vi "AMC_LabVIEW_GUI_Examle_.vi"() -> ()   [LabVIEW 2016]
uses:
  amc_api.lvlib
panel:
  in  "stop":bool
  in  "Tab Control":enum32{"Navigation", "Interface", "About"}(tab)
  out "MoveSignal":bool caption="Moving"
  out "Connected":bool=TRUE
  out "EotrightDetected1":bool caption="Status Eot FWD"
  out "EotLeftDetected1":bool caption="Status Eot BWD"
  out "move out":bool=TRUE caption="Move"
  out "in target range1":bool
  in  "Reset Error":bool
  out "Error":bool
  out "Error Message":string
  in  "Axis Tab Control":enum32{"Operation", "Settings"}(tab)
  out "R [Ohm]":i32
  out "C [nF]":i32
  in  "Single Step\nLeft":bool caption="Open Loop Funktions"
  in  "Single Step\nRight":bool caption="Step(s)"
  in  "Continuous Forward 2":bool caption="Continuous\nForward"
  in  "Endless Left":bool caption="Continuous\nBackward"
  in  "Amplitude [mV]":i32=45
  in  "Frequency [mHz]":i32=1999
  in  "Fixed DC 1":i32 caption="DC Level [mV]"
  in  "Axis 1":bool caption="Closed Loop Functions"
  out "Position":dbl=14701.126 caption="Position [nm]" format="%#_6f"
  out "ReferenceSignal":bool=TRUE
  in  "measureC&R":bool
  in  "Target Position 1":dbl caption="Target position [nm]"
  in  "Move 2":bool
  in  "Positioner":u16(ring)=15 items=["ANGp101", "ANGp50", "ANGt101", "ANGt51", "ANPx101", "ANPx311", "ANPx312", "ANPx321", "ANPx341", "ANPx51", "ANPz101", "ANPz101eXT", "ANPz102", "ANPz51", "ANPz51eXT", "ANR101", "ANR240", "ANR31", "ANR51", "ANRv220", "SNPopenLoop", "SNPxyBottom", "SNPxyTop"]
  in  "Number of steps":i32=1 caption="Number of Steps"
  in  "stop_on_EoT":bool caption="Stop on end of travel"
  in  "Target Range 1":i32 caption="Target Range [nm]"
  in  "Sensor Settings Tab Control":enum32{"NUM only", "RES only"}(tab)
  in  "auto Reset 1":bool=TRUE caption="Auto Reset"
  in  "Reference Auto Update 1":bool=TRUE caption="Auto update reference"
  in  "Configuration upload":path
  in  "Gound on target":bool
  in  "Sensor power":enum16{"0 dB", "-10 dB", "-15 dB", "-20 dB"}(ring)
  in  "auto measure C and R":bool
  in  "Disable Sensor":bool
  in  "Output":bool=TRUE caption="Axis 1"
  out "Output Status":bool=TRUE
  out "status":string
  out "RT Out Tab Control":enum32{"Off", "AquadB", "Trigger"}(tab)
  in  "AqaudB clock 1":i32 caption="AquadB Clock\n[ns], multiple of 40ns"
  in  "AquadB Resolution 1":i32 caption="AquadB\nResolution [nm]"
  in  "Trigger Config":T1
  out "Error 4":bool caption="Error"
  out "Error Message 4":string
  in  "Mode Input":u16(ring) caption="Mode" items=["Trigger (LVDS)"=11, "Trigger (LVTTL)"=10, "Stepper (LVDS)"=9, "Stepper (LVTTL)"=8, "AquadB (LVDS)"=1, "AquadB (LVTTL)"=0, "OFF"=15]
  in  "Loop Mode":u16(ring) caption="Loop mode" items=["closed-loop"=1, "open-loop"=0]
  in  "Steps per pulse":i32 caption="Steps per pulse [Steps]"
  in  "Change per pulse":i32 caption="Change per pulse [u°/nm]"
  in  "Reset Error 4":bool
  in  "Move":bool=TRUE
  in  "Signal mode":enum16{"LVTTL", "LVDS"}(ring)
  in  "RtOutMode":enum16{"Off", "AquadB", "Trigger"}(ring)
  in  "Reset Error 8":bool
  out "Error Message 7":string
  out "Error 7":bool caption="Error"
  out "Sn":string caption="Serial Number"
  out "ip":string="192.168.1.1" caption="IP Adress"
  out "Firmware Version":string
  out "Mac Adress":string
  out "authorized\nStatus":bool
  out "locked\nStatus":bool
  out "device name":string caption="Device Name"
  out "Device type":string="AMC100/NUM"
  out "Features acivated":string[](array[string])
  # "Individual Status Flags"
  # "Closed Loop Functions"
  # "(NUM only)"
  # "Diagnostic Tools (AMC300 only)"
  # "( /PRO Version only )"
  # "( /PRO Version only )"
  # "(AMC300 only)"
  # "Real Time Input"
  # "Real Time Output"
  # "Global Parameters"
  # "Axis 1"
  # "Axis 1"
  # "Device Info"
  # "Device Access"
  # "Features activated"
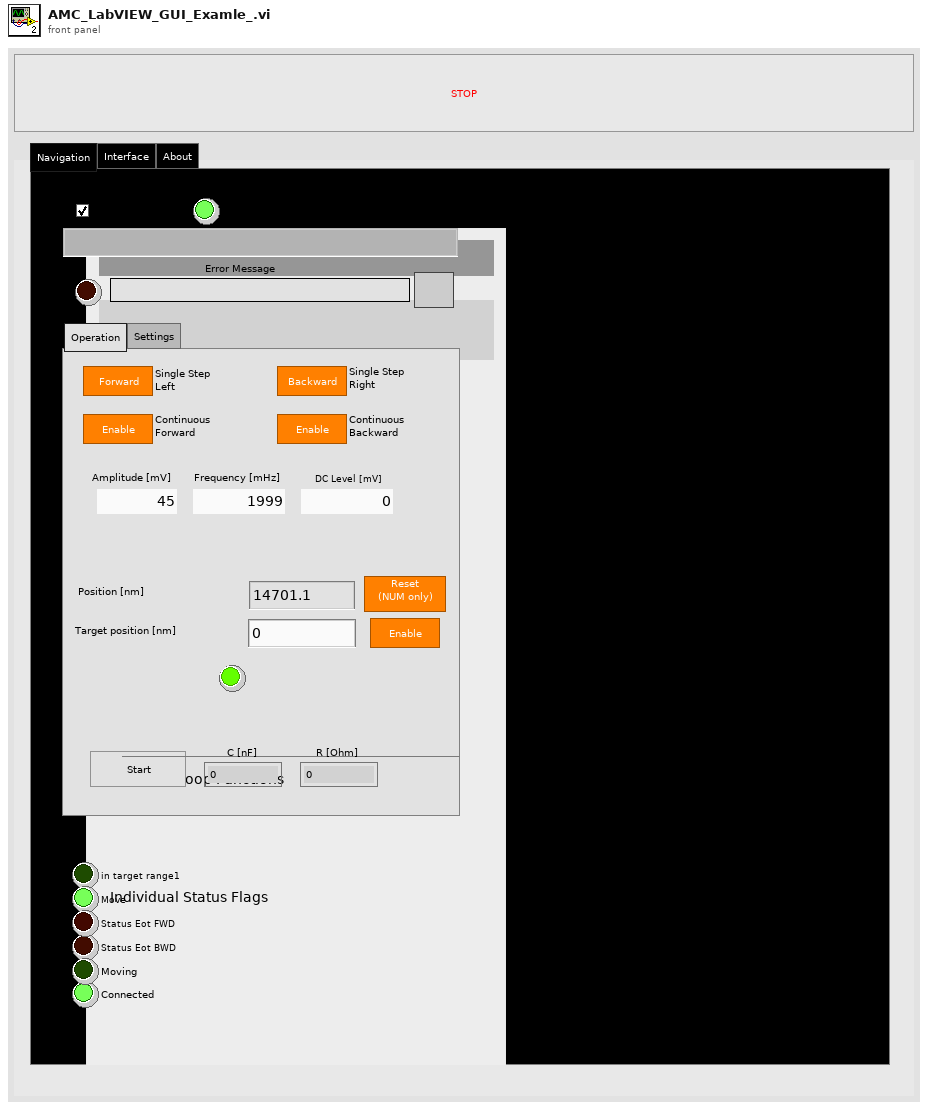
[diagram p1: front panel]
types:
  T1 = cluster{"Position high [nm]":i32, "Position low [nm]":i32, "Trigger polarity":enum16{"Active high", "Active low"}, "Epsilon [nm]":i32}
  T2 = enum8{"Enabled", "Disabled", "Disabled and Grayed Out"}
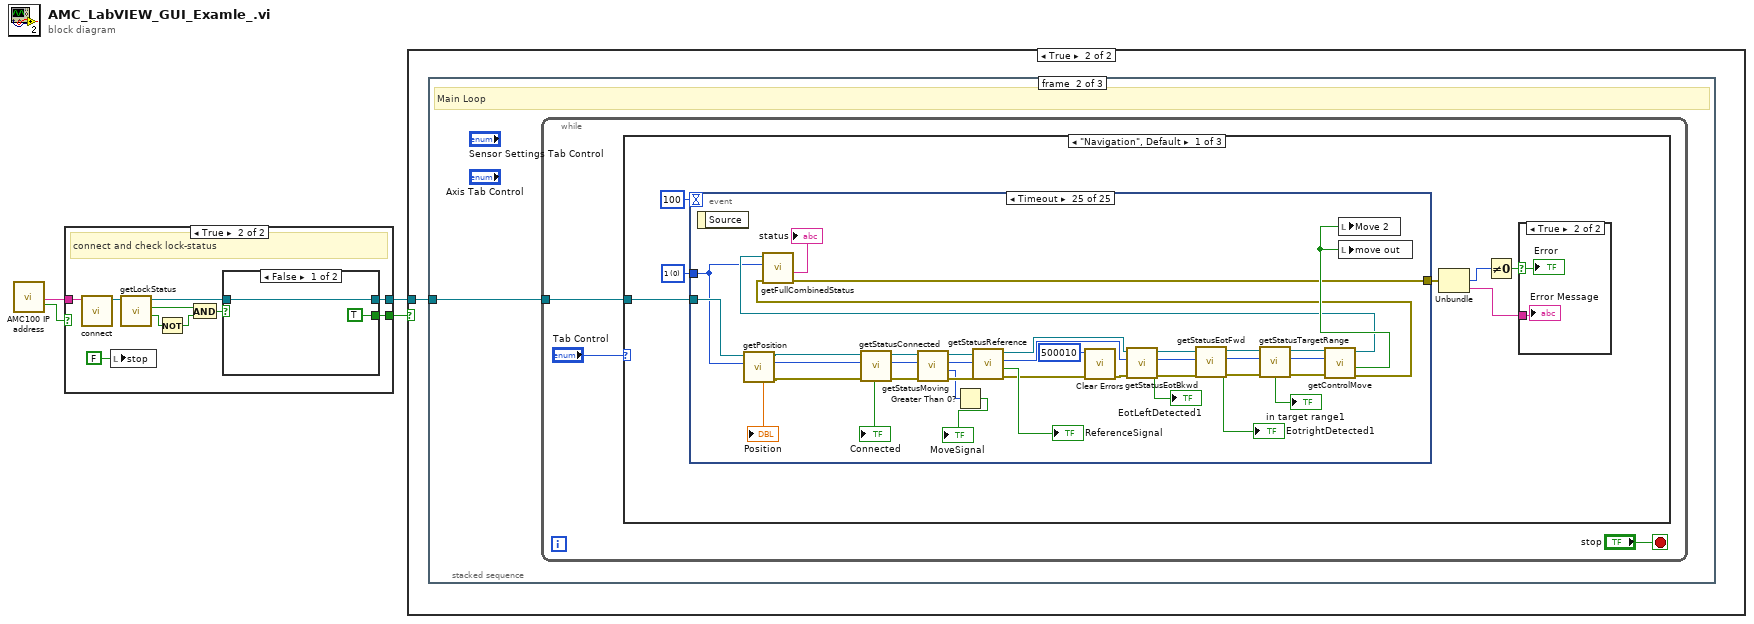
[diagram p0: block diagram]
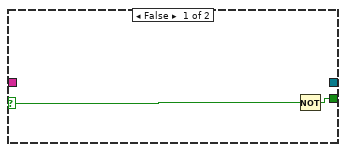
[diagram p2: hidden frame]
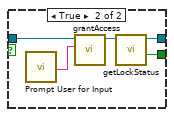
[diagram p3: hidden frame]
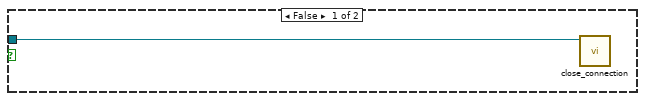
[diagram p4: hidden frame]
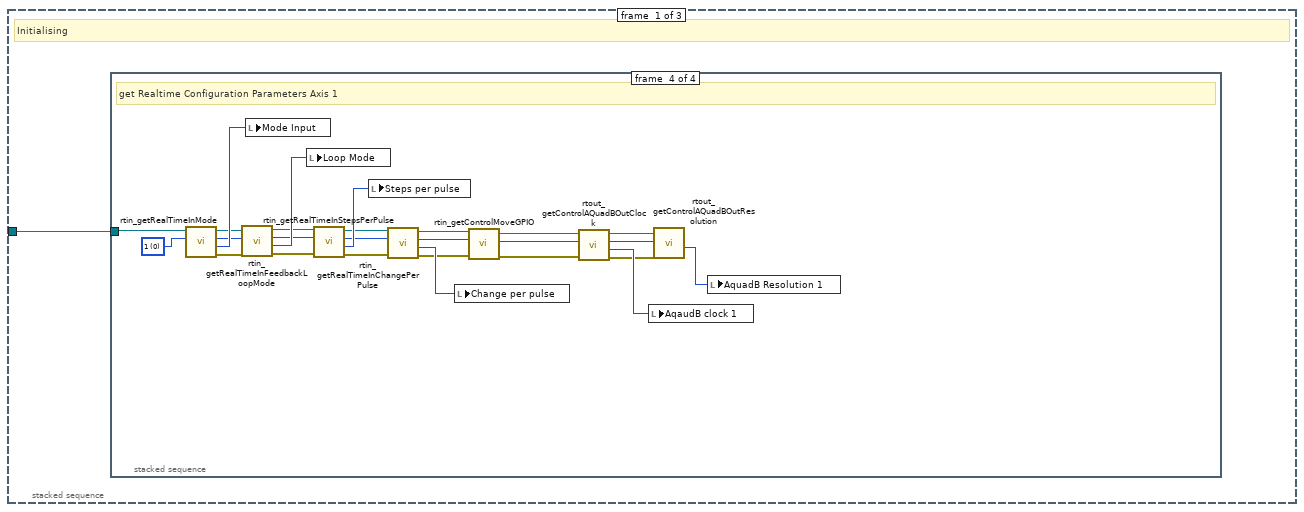
[diagram p5: hidden frame]
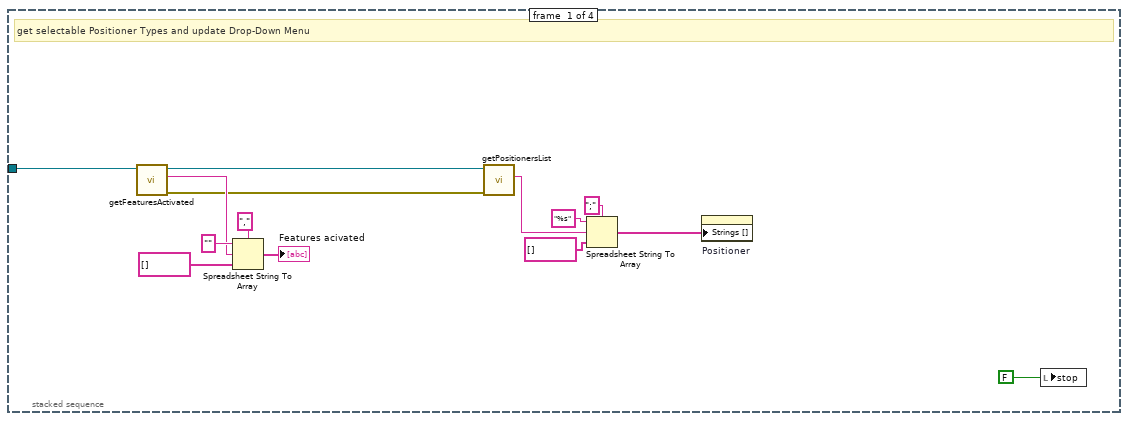
[diagram p6: hidden frame]
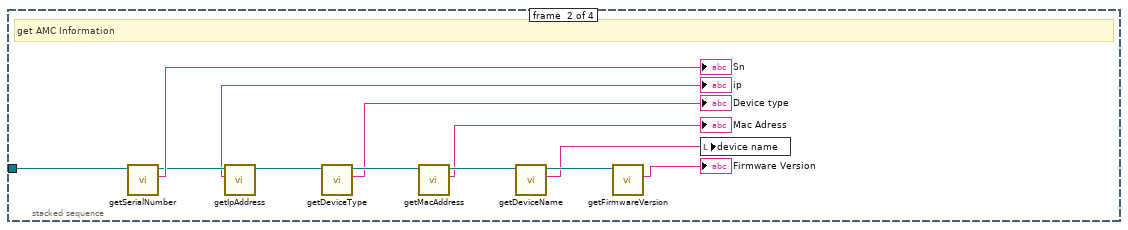
[diagram p7: hidden frame]
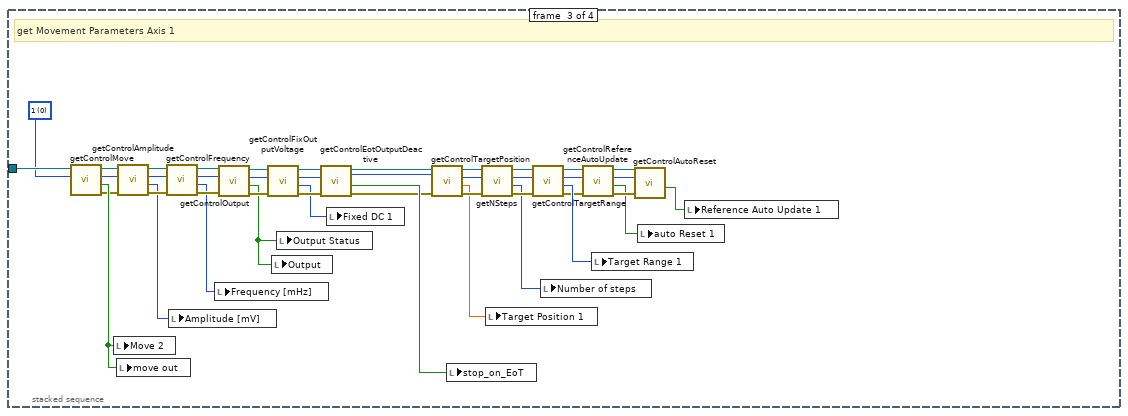
[diagram p8: hidden frame]
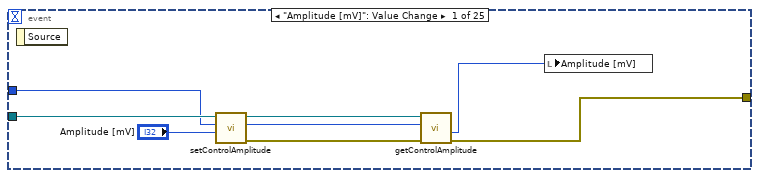
[diagram p10: hidden frame]
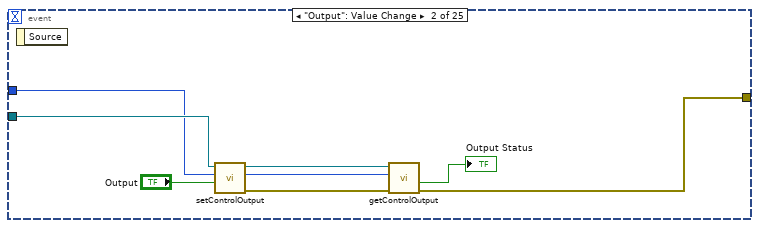
[diagram p11: hidden frame]
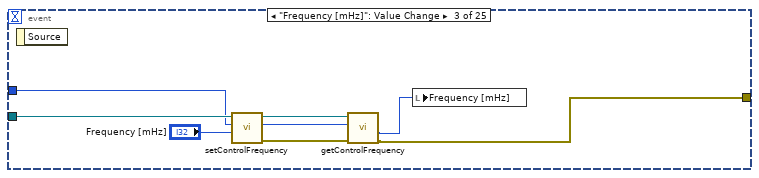
[diagram p12: hidden frame]
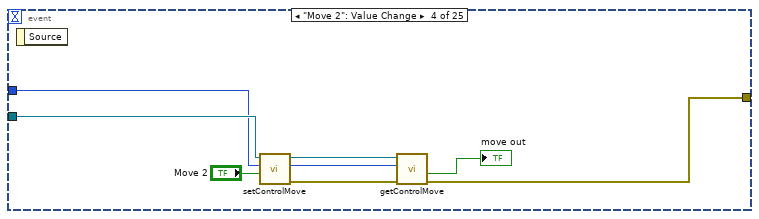
[diagram p13: hidden frame]
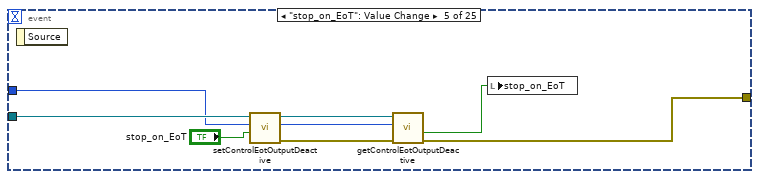
[diagram p14: hidden frame]
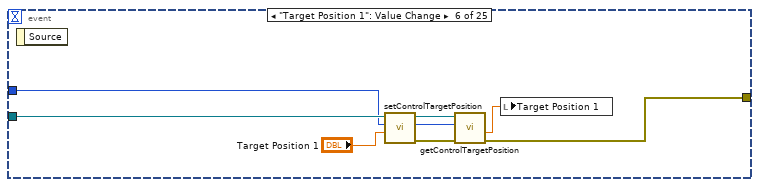
[diagram p15: hidden frame]
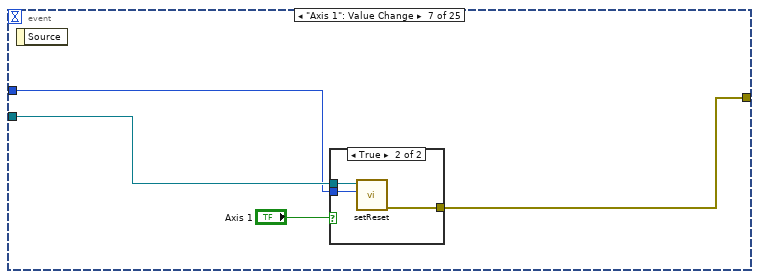
[diagram p16: hidden frame]
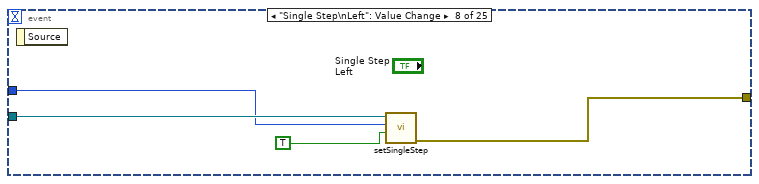
[diagram p18: hidden frame]
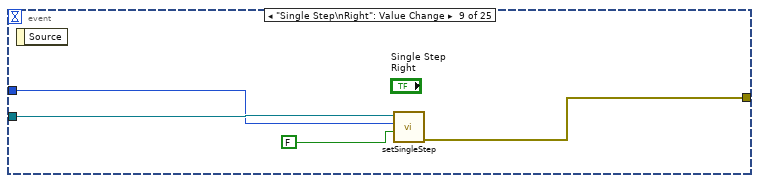
[diagram p19: hidden frame]
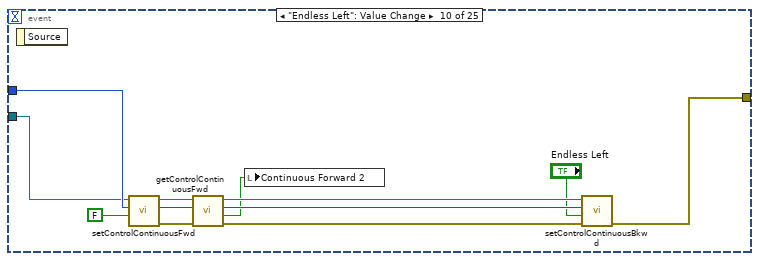
[diagram p20: hidden frame]
diagram:
  n1 = call "AMC100 IP address"() -> ("IP address"=w1:string, "OK"=w2:bool)  [unwired: 17 in, 1 out]
  n2 = case shown="True" w2 {
    selector: w2 -> [w5 _]
    tunnel: [w6 w16] -> w4
    tunnel: [_ w15] -> w3
    tunnel: w1 -> [_ w9]
    frame False {
      n3 = Not(x=w5) -> (.not. x?=w6:bool)
    }
    frame True {
      # "connect and check lock-status"
      n4 = call "connect.vi"("deviceAddress"=w9) -> ("connection ID"=w8:refnum<k5>)  [unwired: 5 in, 1 out]
      n5 = local write "stop"(FALSE ("stop")) -> ()
      n6 = call "getLockStatus.vi"("connection ID"=w8) -> ("authorized"=w11:bool, "locked"=w12:bool, "connection ID out"=w14:refnum<k5>)  [unwired: 7 in, 1 out]
      n7 = Not(x=w11) -> (.not. x?=w10:bool)
      n8 = And(x=w12, y=w10) -> (x .and. y?=w13:bool)
      n9 = case shown="False" w13 {
        tunnel: w14 -> [w18 w23]
        tunnel: [w18 w20] -> w15
        tunnel: [TRUE ("authorized") w19] -> w16
        frame False {
        }
        frame True {
          n10 = call "Prompt User for Input"() -> ("password"=w22:string)  [unwired: 17 in, 2 out]
          n11 = call "grantAccess.vi"("password"=w22, "connection ID"=w23) -> ("connection ID out"=w21:refnum<k5>)  [unwired: 8 in, 1 out]
          n12 = call "getLockStatus.vi"("connection ID"=w21) -> ("authorized"=w19:bool, "connection ID out"=w20:refnum<k5>)  [unwired: 7 in, 2 out]
        }
      }
    }
  }
  n13 = case shown="True" w4 {
    tunnel: w3 -> [w24 w25]
    frame False {
      n14 = call "close_connection.vi"("connection ID"=w24) -> ()  [unwired: 6 in, 1 out]
    }
    frame True {
      n15 = stacked-sequence {
        tunnel: w25 -> [w26 w122 w562]
        frame #0 {
          # "Initialising"
          n16 = stacked-sequence {
            tunnel: w26 -> [w39 w52 w63 w121]
            frame #0 {
              # "get selectable Positioner Types and update Drop-Down Menu"
              n17 = call "getFeaturesActivated.vi"("connection ID"=w39) -> ("error out"=w33:errorcluster, "features"=w36:string, "connection ID out"=w32:refnum<k5>)  [unwired: 8 in]
              n18 = Spreadsheet String To Array(delimiter (Tab)=",", format string="", spreadsheet string=w36, array type (2D Dbl)=string[] []) -> (array=→"Features acivated":string[])
              n19 = call "getPositionersList.vi"("error"=w33, "connection ID"=w32) -> ("PositionersList"=w28:string)  [unwired: 7 in, 2 out]
              n20 = Spreadsheet String To Array(delimiter (Tab)=";", format string="%s", spreadsheet string=w28, array type (2D Dbl)=string[] []) -> (array=w27:string[])
              n21 = property on="Positioner" class="Ring (strict)"("Strings []"=w27) -> ()  [unwired: 2 in, 2 out]
              n22 = local write "stop"(FALSE ("stop")) -> ()
            }
            frame #1 {
              # "get AMC Information"
              n23 = call "getSerialNumber.vi"("connection ID"=w52) -> ("SN"=→"Sn":string, "connection ID out"=w47:refnum<k5>)  [unwired: 8 in, 1 out]
              n24 = call "getIpAddress.vi"("connection ID"=w47) -> ("IP"=→"ip":string, "connection ID out"=w45:refnum<k5>)  [unwired: 8 in, 1 out]
              n25 = call "getDeviceType.vi"("connection ID"=w45) -> ("devicetype"=→"Device type":string, "connection ID out"=w51:refnum<k5>)  [unwired: 8 in, 1 out]
              n26 = call "getMacAddress.vi"("connection ID"=w51) -> ("mac"=→"Mac Adress":string, "connection ID out"=w50:refnum<k5>)  [unwired: 8 in, 1 out]
              n27 = call "getDeviceName.vi"("connection ID"=w50) -> ("name"=w42:string, "connection ID out"=w49:refnum<k5>)  [unwired: 8 in, 1 out]
              n28 = call "getFirmwareVersion.vi"("connection ID"=w49) -> ("FWversion"=→"Firmware Version":string)  [unwired: 8 in, 2 out]
              n29 = local write "device name"(w42) -> ()
            }
            frame #2 {
              w61 = u8 0 items=["1", "2", "3"] ("axis")
              # "get Movement Parameters Axis 1"
              n30 = call "getControlMove.vi"("axis"=w61, "connection ID"=w63) -> ("error out"=w58:errorcluster, "enable"=w59:bool, "axis_out"=w60:i32, "connection ID out"=w62:refnum<k5>)  [unwired: 6 in]
              n31 = local write "Move 2"(w59) -> ()
              n32 = local write "move out"(w59) -> ()
              n33 = call "getControlAmplitude.vi"("error"=w58, "axis"=w60, "connection ID"=w62) -> ("error out"=w93:errorcluster, "amplitude"=w77:i32, "axis_out"=w95:i32, "connection ID out"=w94:refnum<k5>)  [unwired: 5 in]
              n34 = call "getControlFrequency.vi"("error"=w93, "axis"=w95, "connection ID"=w94) -> ("error out"=w90:errorcluster, "frequency"=w76:i32, "axis_out"=w91:i32, "connection ID out"=w92:refnum<k5>)  [unwired: 5 in]
              n35 = local write "Amplitude [mV]"(w77) -> ()
              n36 = local write "Frequency [mHz]"(w76) -> ()
              n37 = call "getControlOutput.vi"("error"=w90, "axis"=w91, "connection ID"=w92) -> ("error out"=w87:errorcluster, "enabled"=w57:bool, "axis_out"=w88:i32, "connection ID out"=w89:refnum<k5>)  [unwired: 5 in]
              n38 = call "getControlFixOutputVoltage.vi"("error"=w87, "axis"=w88, "connection ID"=w89) -> ("error out"=w84:errorcluster, "amplitude_mv"=w75:i32, "axis_out"=w85:i32, "connection ID out"=w86:refnum<k5>)  [unwired: 5 in]
              n39 = local write "Output"(w57) -> ()
              n40 = local write "Output Status"(w57) -> ()
              n41 = call "getControlEotOutputDeactive.vi"("error"=w84, "axis"=w85, "connection ID"=w86) -> ("error out"=w54:errorcluster, "enabled"=w74:bool, "axis_out"=w55:i32, "connection ID out"=w56:refnum<k5>)  [unwired: 5 in]
              n42 = local write "Fixed DC 1"(w75) -> ()
              n43 = call "getControlTargetPosition.vi"("error"=w54, "axis"=w55, "connection ID"=w56) -> ("error out"=w81:errorcluster, "position"=w53:dbl, "axis_out"=w82:i32, "connection ID out"=w83:refnum<k5>)  [unwired: 5 in]
              n44 = local write "stop_on_EoT"(w74) -> ()
              n45 = call "getNSteps.vi"("error"=w81, "axis"=w82, "connection ID"=w83) -> ("error out"=w78:errorcluster, "nbrstep"=w73:i32, "axis_out"=w79:i32, "connection ID out"=w80:refnum<k5>)  [unwired: 5 in]
              n46 = local write "Target Position 1"(w53) -> ()
              n47 = call "getControlTargetRange.vi"("error"=w78, "axis"=w79, "connection ID"=w80) -> ("error out"=w69:errorcluster, "targetrange"=w72:i32, "axis_out"=w70:i32, "connection ID out"=w71:refnum<k5>)  [unwired: 5 in]
              n48 = local write "Number of steps"(w73) -> ()
              n49 = call "getControlReferenceAutoUpdate.vi"("error"=w69, "axis"=w70, "connection ID"=w71) -> ("error out"=w66:errorcluster, "enabled"=w65:bool, "axis_out"=w67:i32, "connection ID out"=w68:refnum<k5>)  [unwired: 5 in]
              n50 = local write "Target Range 1"(w72) -> ()
              n51 = call "getControlAutoReset.vi"("error"=w66, "axis"=w67, "connection ID"=w68) -> ("enabled"=w64:bool)  [unwired: 5 in, 3 out]
              n52 = local write "auto Reset 1"(w65) -> ()
              n53 = local write "Reference Auto Update 1"(w64) -> ()
            }
            frame #3 {
              w99 = u8 0 items=["1", "2", "3"] ("axis")
              # "get Realtime Configuration Parameters Axis 1"
              n54 = call "rtin_getRealTimeInMode.vi"("axis"=w99, "connection ID"=w121) -> ("error out"=w110:errorcluster, "RT_IN_MODE"=w120:i32, "axis_out"=w105:i32, "connection ID out"=w100:refnum<k5>)  [unwired: 6 in]
              n55 = call "rtin_getRealTimeInFeedbackLoopMode.vi"("error"=w110, "axis"=w105, "connection ID"=w100) -> ("error out"=w111:errorcluster, "mode"=w119:i32, "axis_out"=w106:i32, "connection ID out"=w101:refnum<k5>)  [unwired: 5 in]
              n56 = local write "Mode Input"(w120) -> ()
              n57 = local write "Loop Mode"(w119) -> ()
              n58 = call "rtin_getRealTimeInStepsPerPulse.vi"("error"=w111, "axis"=w106, "connection ID"=w101) -> ("error out"=w112:errorcluster, "steps"=w118:i32, "axis_out"=w107:i32, "connection ID out"=w102:refnum<k5>)  [unwired: 5 in]
              n59 = local write "Steps per pulse"(w118) -> ()
              n60 = call "rtin_getRealTimeInChangePerPulse.vi"("error"=w112, "axis"=w107, "connection ID"=w102) -> ("error out"=w113:errorcluster, "resolution"=w117:i32, "axis_out"=w108:i32, "connection ID out"=w103:refnum<k5>)  [unwired: 5 in]
              n61 = local write "Change per pulse"(w117) -> ()
              n62 = call "rtin_getControlMoveGPIO.vi"("error"=w113, "axis"=w108, "connection ID"=w103) -> ("error out"=w96:errorcluster, "axis_out"=w97:i32, "connection ID out"=w98:refnum<k5>)  [unwired: 5 in, 1 out]
              n63 = call "rtout_getControlAQuadBOutClock.vi"("error"=w96, "axis"=w97, "connection ID"=w98) -> ("error out"=w114:errorcluster, "clock_in_ns"=w116:i32, "axis_out"=w109:i32, "connection ID out"=w104:refnum<k5>)  [unwired: 5 in]
              n64 = local write "AqaudB clock 1"(w116) -> ()
              n65 = call "rtout_getControlAQuadBOutResolution.vi"("error"=w114, "axis"=w109, "connection ID"=w104) -> ("resolution"=w115:i32)  [unwired: 5 in, 3 out]
              n66 = local write "AquadB Resolution 1"(w115) -> ()
            }
          }
        }
        frame #1 {
          # "Main Loop"
          n67 = while {
            tunnel: w122 -> [w123]
            stop <- "stop" stop-if-true
            n68 = case shown="\"Navigation\", Default" "Tab Control" {
              tunnel: w123 -> [w132 w379 w547]
              frame "Navigation", Default {
                w131 = u8 0 items=["1", "2", "3"] ("axis in")
                n69 = event shown="[24] Timeout" {
                  selector: _ -> [_ _ _ _ _ _ _ _ _ _ _ _ _ _ _ _ _ _ _ _ _ _ _ _ _]
                  dyn-events: _ -> [_ _ _ _ _ _ _ _ _ _ _ _ _ _ _ _ _ _ _ _ _ _ _ _ _]
                  timeout: 100 -> [_ _ _ _ _ _ _ _ _ _ _ _ _ _ _ _ _ _ _ _ _ _ _ _ _]
                  tunnel: w131 -> [w139 w147 w152 w162 w170 w180 w184 w190 w195 w203 w212 w221 _ w230 w236 w241 w252 w264 w280 w301 w310 w317 w325 w332 w347]
                  tunnel: [w142 w149 w157 w164 w173 w174 w182 w189 w193 w205 w211 w224 _ w228 w239 w247 w255 w263 w273 w304 w305 w320 w328 w331 w342] -> w126
                  tunnel: w132 -> [w140 w148 w154 w163 w171 w181 w185 w191 w196 w197 w213 w223 _ w231 w237 w240 w251 w265 w281 w300 w311 w318 w324 w334 w362]
                  event "Amplitude [mV]": Value Change {
                    n70 = event-data() -> ()  [unwired: 1 in, 1 out]
                    n71 = call "setControlAmplitude.vi"("amplitude"="Amplitude [mV]", "axis"=w139, "connection ID"=w140) -> ("error out"=w137:errorcluster, "axis_out"=w136:i32, "connection ID out"=w135:refnum<k5>)  [unwired: 6 in]
                    n72 = call "getControlAmplitude.vi"("error"=w137, "axis"=w136, "connection ID"=w135) -> ("error out"=w142:errorcluster, "amplitude"=w141:i32)  [unwired: 5 in, 2 out]
                    n73 = local write "Amplitude [mV]"(w141) -> ()
                  }
                  event "Output": Value Change {
                    n74 = event-data() -> ()  [unwired: 1 in, 1 out]
                    n75 = call "setControlOutput.vi"("enable"="Output", "axis"=w147, "connection ID"=w148) -> ("error out"=w145:errorcluster, "axis_out"=w144:i32, "connection ID out"=w143:refnum<k5>)  [unwired: 6 in]
                    n76 = call "getControlOutput.vi"("error"=w145, "axis"=w144, "connection ID"=w143) -> ("error out"=w149:errorcluster, "enabled"=→"Output Status":bool)  [unwired: 5 in, 2 out]
                  }
                  event "Frequency [mHz]": Value Change {
                    n77 = event-data() -> ()  [unwired: 1 in, 1 out]
                    n78 = call "setControlFrequency.vi"("frequency"="Frequency [mHz]", "axis"=w152, "connection ID"=w154) -> ("error out"=w153:errorcluster, "axis_out"=w151:i32)  [unwired: 6 in, 1 out]
                    n79 = call "getControlFrequency.vi"("error"=w153, "axis"=w151, "connection ID"=w154) -> ("error out"=w157:errorcluster, "frequency"=w156:i32)  [unwired: 5 in, 2 out]
                    n80 = local write "Frequency [mHz]"(w156) -> ()
                  }
                  event "Move 2": Value Change {
                    n81 = event-data() -> ()  [unwired: 1 in, 1 out]
                    n82 = call "setControlMove.vi"("enable"="Move 2", "axis"=w162, "connection ID"=w163) -> ("error out"=w160:errorcluster, "axis_out"=w159:i32, "connection ID out"=w158:refnum<k5>)  [unwired: 6 in]
                    n83 = call "getControlMove.vi"("error"=w160, "axis"=w159, "connection ID"=w158) -> ("error out"=w164:errorcluster, "enable"=→"move out":bool)  [unwired: 5 in, 2 out]
                  }
                  event "stop_on_EoT": Value Change {
                    n84 = event-data() -> ()  [unwired: 1 in, 1 out]
                    n85 = call "setControlEotOutputDeactive.vi"("enable"="stop_on_EoT", "axis"=w170, "connection ID"=w171) -> ("error out"=w168:errorcluster, "axis_out"=w166:i32, "connection ID out"=w167:refnum<k5>)  [unwired: 6 in]
                    n86 = call "getControlEotOutputDeactive.vi"("error"=w168, "axis"=w166, "connection ID"=w167) -> ("error out"=w173:errorcluster, "enabled"=w172:bool)  [unwired: 5 in, 2 out]
                    n87 = local write "stop_on_EoT"(w172) -> ()
                  }
                  event "Target Position 1": Value Change {
                    n88 = event-data() -> ()  [unwired: 1 in, 1 out]
                    n89 = call "setControlTargetPosition.vi"("target"="Target Position 1", "axis"=w180, "connection ID"=w181) -> ("error out"=w178:errorcluster, "axis_out"=w177:i32, "connection ID out"=w176:refnum<k5>)  [unwired: 6 in]
                    n90 = call "getControlTargetPosition.vi"("error"=w178, "axis"=w177, "connection ID"=w176) -> ("error out"=w174:errorcluster, "position"=w175:dbl)  [unwired: 5 in, 2 out]
                    n91 = local write "Target Position 1"(w175) -> ()
                  }
                  event "Axis 1": Value Change {
                    n92 = event-data() -> ()  [unwired: 1 in, 1 out]
                    n93 = case shown="True" "Axis 1" {
                      tunnel: [_ w188] -> w182
                      tunnel: w185 -> [_ w187]
                      tunnel: w184 -> [_ w186]
                      frame False {
                      }
                      frame True {
                        n94 = call "setReset.vi"("axis"=w186, "connection ID"=w187) -> ("error out"=w188:errorcluster)  [unwired: 7 in, 2 out]
                      }
                    }
                  }
                  event "Single Step\nLeft": Value Change {
                    n95 = event-data() -> ()  [unwired: 1 in, 1 out]
                    n96 = call "setSingleStep.vi"("backward"=TRUE ("FWD"), "axis"=w190, "connection ID"=w191) -> ("error out"=w189:errorcluster)  [unwired: 6 in, 2 out]
                  }
                  event "Single Step\nRight": Value Change {
                    n97 = event-data() -> ()  [unwired: 1 in, 1 out]
                    n98 = call "setSingleStep.vi"("backward"=FALSE ("FWD"), "axis"=w195, "connection ID"=w196) -> ("error out"=w193:errorcluster)  [unwired: 6 in, 2 out]
                  }
                  event "Endless Left": Value Change {
                    n99 = event-data() -> ()  [unwired: 1 in, 1 out]
                    n100 = call "setControlContinuousFwd.vi"("enable"=FALSE ("continous FWD in"), "axis"=w203, "connection ID"=w197) -> ("error out"=w202:errorcluster, "axis_out"=w201:i32, "connection ID out"=w198:refnum<k5>)  [unwired: 6 in]
                    n101 = call "getControlContinuousFwd.vi"("error"=w202, "axis"=w201, "connection ID"=w198) -> ("error out"=w206:errorcluster, "enabled"=w200:bool, "axis_out"=w207:i32, "connection ID out"=w208:refnum<k5>)  [unwired: 5 in]
                    n102 = local write "Continuous Forward 2"(w200) -> ()
                    n103 = call "setControlContinuousBkwd.vi"("error"=w206, "enable"="Endless Left", "axis"=w207, "connection ID"=w208) -> ("error out"=w205:errorcluster)  [unwired: 5 in, 2 out]
                  }
                  event "Continuous Forward 2": Value Change {
                    n104 = event-data() -> ()  [unwired: 1 in, 1 out]
                    n105 = call "setControlContinuousBkwd.vi"("enable"=FALSE ("continous BWD in"), "axis"=w212, "connection ID"=w213) -> ("error out"=w214:errorcluster, "axis_out"=w215:i32, "connection ID out"=w216:refnum<k5>)  [unwired: 6 in]
                    n106 = call "setControlContinuousFwd.vi"("error"=w214, "enable"="Continuous Forward 2", "axis"=w215, "connection ID"=w216) -> ("error out"=w211:errorcluster)  [unwired: 5 in, 2 out]
                    n107 = local write "Endless Left"(FALSE) -> ()
                  }
                  event "Fixed DC 1": Value Change {
                    n108 = event-data() -> ()  [unwired: 1 in, 1 out]
                    n109 = call "setControlFixOutputVoltage.vi"("amplitude_mv"="Fixed DC 1", "axis"=w221, "connection ID"=w223) -> ("error out"=w218:errorcluster, "axis_out"=w220:i32, "connection ID out"=w219:refnum<k5>)  [unwired: 6 in]
                    n110 = call "getControlFixOutputVoltage.vi"("error"=w218, "axis"=w220, "connection ID"=w219) -> ("error out"=w224:errorcluster, "amplitude_mv"=w225:i32)  [unwired: 5 in, 2 out]
                    n111 = local write "Fixed DC 1"(w225) -> ()
                  }
                  event "Reset Error": Value Change {
                    n112 = event-data() -> ()  [unwired: 1 in, 1 out]
                    n113 = local write "Error Message"("" ("Error Message")) -> ()
                    n114 = local write "Error"(FALSE ("Error")) -> ()
                  }
                  event "Positioner": Value Change {
                    n115 = event-data() -> ()  [unwired: 1 in, 1 out]
                    n116 = property on="Positioner" class="Ring (strict)"() -> ("RingText.Text"=w229:string)  [unwired: 2 in, 2 out]
                    n117 = call "setActorParametersByName.vi"("actorname"=w229, "axis"=w230, "connection ID"=w231) -> ("error out"=w228:errorcluster)  [unwired: 6 in, 2 out]
                  }
                  event "Target Range 1": Value Change {
                    n118 = event-data() -> ()  [unwired: 1 in, 1 out]
                    n119 = call "setControlTargetRange.vi"("range"="Target Range 1", "axis"=w236, "connection ID"=w237) -> ("error out"=w234:errorcluster, "axis_out"=w232:i32, "connection ID out"=w233:refnum<k5>)  [unwired: 6 in]
                    n120 = call "getControlTargetRange.vi"("error"=w234, "axis"=w232, "connection ID"=w233) -> ("error out"=w239:errorcluster, "targetrange"=w238:i32)  [unwired: 5 in, 2 out]
                    n121 = local write "Target Range 1"(w238) -> ()
                  }
                  event "auto Reset 1": Value Change {
                    n122 = event-data() -> ()  [unwired: 1 in, 1 out]
                    n123 = call "setControlAutoReset.vi"("enable"="auto Reset 1", "axis"=w241, "connection ID"=w240) -> ("error out"=w242:errorcluster, "axis_out"=w243:i32, "connection ID out"=w244:refnum<k5>)  [unwired: 6 in]
                    n124 = call "getControlAutoReset.vi"("error"=w242, "axis"=w243, "connection ID"=w244) -> ("error out"=w247:errorcluster, "enabled"=w246:bool)  [unwired: 5 in, 2 out]
                    n125 = local write "auto Reset 1"(w246) -> ()
                  }
                  event "Reference Auto Update 1": Value Change {
                    n126 = event-data() -> ()  [unwired: 1 in, 1 out]
                    n127 = call "setControlReferenceAutoUpdate.vi"("enable"="Reference Auto Update 1", "axis"=w252, "connection ID"=w251) -> ("error out"=w248:errorcluster, "axis_out"=w250:i32, "connection ID out"=w249:refnum<k5>)  [unwired: 6 in]
                    n128 = call "getControlReferenceAutoUpdate.vi"("error"=w248, "axis"=w250, "connection ID"=w249) -> ("error out"=w255:errorcluster, "enabled"=w254:bool)  [unwired: 5 in, 2 out]
                    n129 = local write "Reference Auto Update 1"(w254) -> ()
                  }
                  event "Configuration upload": Value Change {
                    n130 = event-data() -> ()  [unwired: 1 in, 1 out]
                    n131 = Open/Create/Replace File(file path (use dialog)="Configuration upload") -> (refnum out=w259:refnum<file>, error out=w262:errorcluster)  [unwired: 5 in, 1 out]
                    n132 = Read from Text File(file (use dialog)=w259, error in=w262) -> (refnum out=w260:refnum<file>, text=w257:string, error out=w261:errorcluster)  [unwired: 2 in, 1 out]
                    n133 = Close File(refnum=w260, error in=w261) -> (error out=w256:errorcluster)  [unwired: 1 out]
                    n134 = case shown="Error" w256 {
                      selector: w256 -> [_ w270]
                      tunnel: w265 -> [w269 _]
                      tunnel: w264 -> [w268 _]
                      tunnel: [w267 w270] -> w263
                      tunnel: w257 -> [w266 _]
                      frame No Error {
                        n135 = call "setConfigurationFile.vi"("content"=w266, "axis"=w268, "connection ID"=w269) -> ("error out"=w267:errorcluster)  [unwired: 6 in, 2 out]
                      }
                      frame Error {
                      }
                    }
                  }
                  event "measureC&R": Value Change {
                    n136 = event-data() -> ()  [unwired: 1 in, 1 out]
                    n137 = flat-sequence {
                      tunnel: w281 -> [w286]
                      tunnel: w280 -> [w285]
                      tunnel: [w284] -> w279
                      tunnel: [w283] -> w278
                      tunnel: [w282] -> w277
                      tunnel: w279 -> [w290]
                      tunnel: w278 -> [w289]
                      tunnel: w277 -> [w288]
                      tunnel: [w290] -> w276
                      tunnel: [w289] -> w275
                      tunnel: [w288] -> w274
                      tunnel: w276 -> [w296]
                      tunnel: w275 -> [w293]
                      tunnel: w274 -> [w294]
                      tunnel: [w295] -> w273
                      tunnel: [w292] -> w272
                      tunnel: [w291] -> w271
                      frame #0 {
                        n138 = call "startDiagnostic.vi"("axis"=w285, "connection ID"=w286) -> ("error out"=w284:errorcluster, "axis_out"=w283:i32, "connection ID out"=w282:refnum<k5>)  [unwired: 7 in]
                      }
                      frame #1 {
                        n139 = Wait (ms)(milliseconds to wait=u32 5000) -> ()  [unwired: 1 out]
                      }
                      frame #2 {
                        n140 = call "getDiagnosticResults.vi"("connection ID"=w294, "axis"=w293, "error"=w296) -> ("capacity"=w292:i32, "resistance"=w291:i32, "error out"=w295:errorcluster)  [unwired: 12 in, 2 out]
                      }
                    }
                    "C [nF]" <- w272
                    "R [Ohm]" <- w271
                  }
                  event "Gound on target": Value Change {
                    n141 = event-data() -> ()  [unwired: 1 in, 1 out]
                    n142 = call "setGroundAxisAutoOnTarget.vi"("enabled"="Gound on target", "axis"=w301, "connection ID"=w300) -> ("error out"=w297:errorcluster, "axis_out"=w299:i32, "connection ID out"=w298:refnum<k5>)  [unwired: 6 in]
                    n143 = call "getGroundAxisAutoOnTarget.vi"("error"=w297, "axis"=w299, "connection ID"=w298) -> ("error out"=w304:errorcluster, "value"=w303:bool)  [unwired: 5 in, 2 out]
                    n144 = local write "Gound on target"(w303) -> ()
                  }
                  event "auto measure C and R": Value Change {
                    n145 = event-data() -> ()  [unwired: 1 in, 1 out]
                    n146 = call "setAutoMeasure.vi"("enable"="auto measure C and R", "axis"=w310, "connection ID"=w311) -> ("error out"=w309:errorcluster, "axis_out"=w307:i32, "connection ID out"=w308:refnum<k5>)  [unwired: 6 in]
                    n147 = call "getAutoMeasure.vi"("error"=w309, "axis"=w307, "connection ID"=w308) -> ("error out"=w305:errorcluster, "enable"=w306:bool)  [unwired: 5 in, 2 out]
                    n148 = local write "auto measure C and R"(w306) -> ()
                  }
                  event "Sensor power": Value Change {
                    n149 = event-data() -> ()  [unwired: 1 in, 1 out]
                    n150 = call "setChainGain.vi"("gainconfig"="Sensor power", "axis"=w317, "connection ID"=w318) -> ("error out"=w313:errorcluster, "axis_out"=w315:i32, "connection ID out"=w314:refnum<k5>)  [unwired: 6 in]
                    n151 = call "getChainGain.vi"("error"=w313, "axis"=w315, "connection ID"=w314) -> ("error out"=w320:errorcluster, "gaincoeff"=w319:i32)  [unwired: 5 in, 2 out]
                    n152 = local write "Sensor power"(w319) -> ()
                  }
                  event "Disable Sensor": Value Change {
                    n153 = event-data() -> ()  [unwired: 1 in, 1 out]
                    n154 = Not(x="Disable Sensor") -> (.not. x?=w326:bool)
                    n155 = call "setSensorEnabled.vi"("value"=w326, "axis"=w325, "connection ID"=w324) -> ("error out"=w323:errorcluster, "axis_out"=w321:i32, "connection ID out"=w322:refnum<k5>)  [unwired: 6 in]
                    n156 = call "getSensorEnabled.vi"("error"=w323, "axis"=w321, "connection ID"=w322) -> ("error out"=w328:errorcluster, "value"=w327:bool)  [unwired: 5 in, 2 out]
                    n157 = Not(x=w327) -> (.not. x?=w329:bool)
                    n158 = local write "Disable Sensor"(w329) -> ()
                  }
                  event "Number of steps": Value Change {
                    n159 = event-data() -> ()  [unwired: 1 in, 1 out]
                    n160 = call "writeNSteps.vi"("step"="Number of steps", "axis"=w332, "connection ID"=w334) -> ("error out"=w331:errorcluster)  [unwired: 6 in, 2 out]
                  }
                  event Timeout {
                    n161 = event-data() -> ()  [unwired: 1 in, 1 out]
                    n162 = call "getPosition.vi"("axis"=w347, "connection ID"=w362) -> ("error out"=w341:errorcluster, "position"=→"Position":dbl, "axis_out"=w340:i32, "connection ID out"=w339:refnum<k5>)  [unwired: 6 in]
                    n163 = call "getStatusConnected.vi"("error"=w341, "axis"=w340, "connection ID"=w339) -> ("error out"=w357:errorcluster, "connected"=→"Connected":bool, "axis_out"=w371:i32, "connection ID out"=w372:refnum<k5>)  [unwired: 5 in]
                    n164 = call "getStatusMoving.vi"("error"=w357, "axis"=w371, "connection ID"=w372) -> ("error out"=w356:errorcluster, "status"=w344:i32, "axis_out"=w369:i32, "connection ID out"=w370:refnum<k5>)  [unwired: 5 in]
                    n165 = Greater Than 0?(x=w344) -> (x > 0?=→"MoveSignal":bool)
                    n166 = call "getStatusReference.vi"("error"=w356, "axis"=w369, "connection ID"=w370) -> ("error out"=w337:errorcluster, "valid"=→"ReferenceSignal":bool, "axis_out"=w367:i32, "connection ID out"=w368:refnum<k5>)  [unwired: 5 in]
                    n167 = call <vilib>:"Clear Errors.vi"("error in (no error)"=w337, "specific error code to clear (0: all)"=500010) -> ("error out"=w336:errorcluster)  [unwired: 4 in, 1 out]
                    n168 = call "getStatusEotBkwd.vi"("error"=w336, "axis"=w367, "connection ID"=w368) -> ("error out"=w355:errorcluster, "detected"=→"EotLeftDetected1":bool, "axis_out"=w365:i32, "connection ID out"=w366:refnum<k5>)  [unwired: 5 in]
                    n169 = call "getStatusEotFwd.vi"("error"=w355, "axis"=w365, "connection ID"=w366) -> ("error out"=w354:errorcluster, "detected"=→"EotrightDetected1":bool, "axis_out"=w363:i32, "connection ID out"=w364:refnum<k5>)  [unwired: 5 in]
                    n170 = call "getStatusTargetRange.vi"("error"=w354, "axis"=w363, "connection ID"=w364) -> ("error out"=w351:errorcluster, "in_range"=→"in target range1":bool, "axis_out"=w352:i32, "connection ID out"=w353:refnum<k5>)  [unwired: 5 in]
                    n171 = call "getControlMove.vi"("error"=w351, "axis"=w352, "connection ID"=w353) -> ("error out"=w346:errorcluster, "enable"=w350:bool, "connection ID out"=w348:refnum<k5>)  [unwired: 5 in, 1 out]
                    n172 = call "getFullCombinedStatus.vi"("error"=w346, "axis"=w347, "connection ID"=w348) -> ("error out"=w342:errorcluster, "status_str"=→"status":string)  [unwired: 5 in, 2 out]
                    n173 = local write "Move 2"(w350) -> ()
                    n174 = local write "move out"(w350) -> ()
                  }
                }
                n175 = Unbundle(w126) -> ("code"=w128:i32, "source"=w129:string)  [unwired: 1 out]
                n176 = Not Equal To 0?(x=w128) -> (x != 0?=w127:bool)
                n177 = case shown="True" w127 {
                  selector: w127 -> [_ w133]
                  tunnel: w129 -> [_ w134]
                  frame False {
                  }
                  frame True {
                    "Error Message" <- w134
                    "Error" <- w133
                  }
                }
              }
              frame "Interface" {
                w378 = u8 0 items=["1", "2", "3"] ("axis in")
                n178 = event shown="[2] \"Loop Mode\": Value Change" {
                  selector: _ -> [_ _ _ _ _ _ _ _ _ _ _ _]
                  dyn-events: _ -> [_ _ _ _ _ _ _ _ _ _ _ _]
                  timeout: 100 -> [_ _ _ _ _ _ _ _ _ _ _ _]
                  tunnel: w378 -> [w385 w460 w463 w474 w478 w490 w498 w506 _ w520 w538 _]
                  tunnel: [w384 w459 w469 w476 w484 w492 w501 w509 w515 w522 w530 _] -> w375
                  tunnel: w379 -> [w386 w461 w464 w475 w480 w491 w499 w507 w514 w521 w539 _]
                  event Timeout {
                    n179 = event-data() -> ()  [unwired: 1 in, 1 out]
                    n180 = stacked-sequence {
                      tunnel: w386 -> [w398 w429]
                      tunnel: w385 -> [w397 w426]
                      tunnel: [w390 _] -> w383
                      tunnel: [_ w433] -> w382
                      frame #0 {
                        # "get RT Input\nSettings"
                        n181 = call "rtin_getRealTimeInStepsPerPulse.vi"("axis"=w397, "connection ID"=w398) -> ("error out"=w393:errorcluster, "steps"=w399:i32, "axis_out"=w389:i32, "connection ID out"=w396:refnum<k5>)  [unwired: 6 in]
                        n182 = call "rtin_getRealTimeInChangePerPulse.vi"("error"=w393, "axis"=w389, "connection ID"=w396) -> ("error out"=w392:errorcluster, "resolution"=w400:i32, "axis_out"=w388:i32, "connection ID out"=w395:refnum<k5>)  [unwired: 5 in]
                        n183 = local write "Steps per pulse"(w399) -> ()
                        n184 = call "rtin_getControlMoveGPIO.vi"("error"=w392, "axis"=w388, "connection ID"=w395) -> ("error out"=w391:errorcluster, "enable"=w401:bool, "axis_out"=w387:i32, "connection ID out"=w394:refnum<k5>)  [unwired: 5 in]
                        n185 = local write "Change per pulse"(w400) -> ()
                        n186 = call "rtin_getRealTimeInMode.vi"("error"=w391, "axis"=w387, "connection ID"=w394) -> ("error out"=w407:errorcluster, "RT_IN_MODE"=w410:i32, "axis_out"=w408:i32, "connection ID out"=w409:refnum<k5>)  [unwired: 5 in]
                        n187 = local write "Move"(w401) -> ()
                        n188 = Equal?(x=w410, y=15) -> (x = y?=w412:bool)
                        n189 = call "rtin_getRealTimeInFeedbackLoopMode.vi"("error"=w407, "axis"=w408, "connection ID"=w409) -> ("error out"=w390:errorcluster, "mode"=w402:i32)  [unwired: 5 in, 2 out]
                        n190 = local write "Loop Mode"(w402) -> ()
                        n191 = local write "Mode Input"(w410) -> ()
                        n192 = Equal To 0?(x=w402) -> (x = 0?=w411:bool)
                        n193 = case shown="False" w412 {
                          tunnel: w411 -> [w418 _]
                          tunnel: [w417 w423] -> w406
                          tunnel: [w416 w423] -> w405
                          tunnel: [w415 w423] -> w404
                          tunnel: [w414 w423] -> w403
                          frame False {
                            # "RT Input ON"
                            n194 = case shown="True" w418 {
                              tunnel: [w419 w422] -> w417
                              tunnel: [w419 w421] -> w416
                              tunnel: [T2."Disabled and Grayed Out" ("Disabled") w422] -> w414
                              tunnel: [w419 w421] -> w415
                              frame False {
                                w419 = T2."Enabled" ("Disabled")
                                # "closed-loop Mode"
                              }
                              frame True {
                                w422 = T2."Enabled" ("Disabled")
                                w421 = T2."Disabled and Grayed Out" ("Disabled")
                                # "open-loop Mode"
                              }
                            }
                          }
                          frame True {
                            w423 = T2."Disabled and Grayed Out" ("Disabled")
                            # "RT Input OFF"
                          }
                        }
                        n195 = property on="Loop Mode" class="Ring (strict)"("DisabledEnum"=w406) -> ()  [unwired: 2 in, 2 out]
                        n196 = property on="Move" class="Bool (strict)"("DisabledEnum"=w404) -> ()  [unwired: 2 in, 2 out]
                        n197 = property on="Change per pulse" class="DigNum (strict)"("DisabledEnum"=w405) -> ()  [unwired: 2 in, 2 out]
                        n198 = property on="Steps per pulse" class="DigNum (strict)"("DisabledEnum"=w403) -> ()  [unwired: 2 in, 2 out]
                      }
                      frame #1 {
                        # "get RT Output\nSettings"
                        n199 = call "rtout_getSignalMode.vi"("connection ID"=w429) -> ("error out"=w427:errorcluster, "mode"=w424:i32, "connection ID out"=w428:refnum<k5>)  [unwired: 8 in]
                        n200 = call "rtout_getMode.vi"("error"=w427, "axis"=w426, "connection ID"=w428) -> ("error out"=w430:errorcluster, "RT_OUT_MODE"=w425:i32, "axis_out"=w431:i32, "connection ID out"=w432:refnum<k5>)  [unwired: 5 in]
                        n201 = local write "Signal mode"(w424) -> ()
                        n202 = case shown="2" w425 {
                          tunnel: w432 -> [_ w442 w453]
                          tunnel: w430 -> [w434 w441 w452]
                          tunnel: w431 -> [_ w437 w445]
                          tunnel: [w434 w435 w451] -> w433
                          frame 0, Default {
                          }
                          frame 1 {
                            n203 = call "rtout_getControlAQuadBOutClock.vi"("error"=w441, "axis"=w437, "connection ID"=w442) -> ("error out"=w440:errorcluster, "clock_in_ns"=w438:i32, "axis_out"=w436:i32, "connection ID out"=w439:refnum<k5>)  [unwired: 5 in]
                            n204 = call "rtout_getControlAQuadBOutResolution.vi"("error"=w440, "axis"=w436, "connection ID"=w439) -> ("error out"=w435:errorcluster, "resolution"=w443:i32)  [unwired: 5 in, 2 out]
                            n205 = local write "AqaudB clock 1"(w438) -> ()
                            n206 = local write "AquadB Resolution 1"(w443) -> ()
                          }
                          frame 2 {
                            n207 = call "rtout_getTriggerConfig.vi"("connection ID"=w453, "axis"=w445, "error"=w452) -> ("polarity"=w444:i32, "higher"=w447:i32, "lower"=w448:i32, "epsilon"=w449:i32, "error out"=w451:errorcluster)  [unwired: 10 in, 2 out]
                            n208 = Bundle(cluster=T1 {"Position high [nm]"=0, "Position low [nm]"=0, "Trigger polarity"=enum."Active high", "Epsilon [nm]"=0} ("Trigger Config"), "Position high [nm]"=w447, "Position low [nm]"=w448, "Trigger polarity"=w444, "Epsilon [nm]"=w449) -> (w446:T1)
                            n209 = local write "Trigger Config"(w446) -> ()
                          }
                        }
                        n210 = local write "RT Out Tab Control"(w425) -> ()
                        n211 = local write "RtOutMode"(w425) -> ()
                      }
                    }
                    n212 = Merge Errors(w383, w382) -> (w384:errorcluster)
                  }
                  event "Mode Input": Value Change {
                    n213 = event-data() -> ()  [unwired: 1 in, 1 out]
                    n214 = call "rtin_setRealTimeInMode.vi"("RT_IN_MODE"="Mode Input", "axis"=w460, "connection ID"=w461) -> ("error out"=w455:errorcluster, "axis_out"=w456:i32, "connection ID out"=w457:refnum<k5>)  [unwired: 6 in]
                    n215 = local write "Mode Input"("Mode Input") -> ()
                    n216 = call "rtin_getRealTimeInFeedbackLoopMode.vi"("error"=w455, "axis"=w456, "connection ID"=w457) -> ("error out"=w459:errorcluster, "mode"=w458:i32)  [unwired: 5 in, 2 out]
                    n217 = local write "Loop Mode"(w458) -> ()
                  }
                  event "Loop Mode": Value Change {
                    n218 = event-data() -> ()  [unwired: 1 in, 1 out]
                    n219 = call "rtin_setRealTimeInFeedbackLoopMode.vi"("mode"="Loop Mode", "axis"=w463, "connection ID"=w464) -> ("error out"=w467:errorcluster, "axis_out"=w466:i32, "connection ID out"=w465:refnum<k5>)  [unwired: 6 in]
                    n220 = call "rtin_getRealTimeInFeedbackLoopMode.vi"("error"=w467, "axis"=w466, "connection ID"=w465) -> ("error out"=w469:errorcluster, "mode"=w468:i32)  [unwired: 5 in, 2 out]
                    n221 = local write "Loop Mode"(w468) -> ()
                  }
                  event "Steps per pulse": Value Change {
                    n222 = event-data() -> ()  [unwired: 1 in, 1 out]
                    n223 = call "rtin_setRealTimeInStepsPerPulse.vi"("steps"="Steps per pulse", "axis"=w474, "connection ID"=w475) -> ("error out"=w470:errorcluster, "axis_out"=w472:i32, "connection ID out"=w471:refnum<k5>)  [unwired: 6 in]
                    n224 = call "rtin_getRealTimeInStepsPerPulse.vi"("error"=w470, "axis"=w472, "connection ID"=w471) -> ("error out"=w476:errorcluster, "steps"=w477:i32)  [unwired: 5 in, 2 out]
                    n225 = local write "Steps per pulse"(w477) -> ()
                  }
                  event "Change per pulse": Value Change {
                    n226 = event-data() -> ()  [unwired: 1 in, 1 out]
                    n227 = call "rtin_setRealTimeInChangePerPulse.vi"("delta"="Change per pulse", "axis"=w478, "connection ID"=w480) -> ("error out"=w481:errorcluster, "axis_out"=w482:i32, "connection ID out"=w483:refnum<k5>)  [unwired: 6 in]
                    n228 = call "rtin_getRealTimeInChangePerPulse.vi"("error"=w481, "axis"=w482, "connection ID"=w483) -> ("error out"=w484:errorcluster, "resolution"=w485:i32)  [unwired: 5 in, 2 out]
                    n229 = local write "Change per pulse"(w485) -> ()
                  }
                  event "Move": Value Change {
                    n230 = event-data() -> ()  [unwired: 1 in, 1 out]
                    n231 = call "rtin_setControlMoveGPIO.vi"("enable"="Move", "axis"=w490, "connection ID"=w491) -> ("error out"=w489:errorcluster, "axis_out"=w488:i32, "connection ID out"=w487:refnum<k5>)  [unwired: 6 in]
                    n232 = call "rtin_getControlMoveGPIO.vi"("error"=w489, "axis"=w488, "connection ID"=w487) -> ("error out"=w492:errorcluster, "enable"=w493:bool)  [unwired: 5 in, 2 out]
                    n233 = local write "Move"(w493) -> ()
                  }
                  event "AqaudB clock 1": Value Change {
                    n234 = event-data() -> ()  [unwired: 1 in, 1 out]
                    n235 = call "rtout_setControlAQuadBOutClock.vi"("clock"="AqaudB clock 1", "axis"=w498, "connection ID"=w499) -> ("error out"=w494:errorcluster, "axis_out"=w496:i32, "connection ID out"=w495:refnum<k5>)  [unwired: 6 in]
                    n236 = call "rtout_getControlAQuadBOutClock.vi"("error"=w494, "axis"=w496, "connection ID"=w495) -> ("error out"=w501:errorcluster, "clock_in_ns"=w500:i32)  [unwired: 5 in, 2 out]
                    n237 = local write "AqaudB clock 1"(w500) -> ()
                  }
                  event "AquadB Resolution 1": Value Change {
                    n238 = event-data() -> ()  [unwired: 1 in, 1 out]
                    n239 = call "rtout_setControlAQuadBOutResolution.vi"("resolution"="AquadB Resolution 1", "axis"=w506, "connection ID"=w507) -> ("error out"=w502:errorcluster, "axis_out"=w504:i32, "connection ID out"=w503:refnum<k5>)  [unwired: 6 in]
                    n240 = call "rtout_getControlAQuadBOutResolution.vi"("error"=w502, "axis"=w504, "connection ID"=w503) -> ("error out"=w509:errorcluster, "resolution"=w508:i32)  [unwired: 5 in, 2 out]
                    n241 = local write "AquadB Resolution 1"(w508) -> ()
                  }
                  event "Signal mode": Value Change {
                    n242 = event-data() -> ()  [unwired: 1 in, 6 out]
                    n243 = call "rtout_setSignalMode.vi"("mode"="Signal mode", "connection ID"=w514) -> ("error out"=w511:errorcluster, "connection ID out"=w512:refnum<k5>)  [unwired: 8 in]
                    n244 = call "rtout_getSignalMode.vi"("error"=w511, "connection ID"=w512) -> ("error out"=w515:errorcluster, "mode"=w510:i32)  [unwired: 7 in, 1 out]
                    n245 = local write "Signal mode"(w510) -> ()
                  }
                  event "RtOutMode": Value Change {
                    n246 = event-data() -> ()  [unwired: 1 in, 1 out]
                    n247 = call "rtout_setMode.vi"("RT_OUT_MODE"="RtOutMode", "axis"=w520, "connection ID"=w521) -> ("error out"=w518:errorcluster, "axis_out"=w517:i32, "connection ID out"=w516:refnum<k5>)  [unwired: 6 in]
                    n248 = call "rtout_getMode.vi"("error"=w518, "axis"=w517, "connection ID"=w516) -> ("error out"=w522:errorcluster, "RT_OUT_MODE"=w523:i32)  [unwired: 5 in, 2 out]
                    "RT Out Tab Control" <- w523
                    n249 = local write "RtOutMode"(w523) -> ()
                  }
                  event "Trigger Config": Value Change {
                    n250 = event-data() -> ()  [unwired: 1 in, 1 out]
                    n251 = Unbundle("Trigger Config") -> ("Position high [nm]"=w535:i32, "Position low [nm]"=w534:i32, "Trigger polarity"=w533:enum16{"Active high", "Active low"}, "Epsilon [nm]"=w532:i32)
                    n252 = call "rtout_setTriggerConfig.vi"("connection ID"=w539, "axis"=w538, "higher"=w535, "lower"=w534, "epsilon"=w532, "polarity"=w533) -> ("connection ID out"=w529:refnum<k5>, "axis_out"=w528:i32, "error out"=w531:errorcluster)  [unwired: 11 in]
                    n253 = call "rtout_getTriggerConfig.vi"("connection ID"=w529, "axis"=w528, "error"=w531) -> ("polarity"=w524:i32, "higher"=w525:i32, "lower"=w526:i32, "epsilon"=w527:i32, "error out"=w530:errorcluster)  [unwired: 10 in, 2 out]
                    n254 = Bundle(cluster=T1 {"Position high [nm]"=0, "Position low [nm]"=0, "Trigger polarity"=enum."Active high", "Epsilon [nm]"=0} ("Trigger Config"), "Position high [nm]"=w525, "Position low [nm]"=w526, "Trigger polarity"=w524, "Epsilon [nm]"=w527) -> (w536:T1)
                    n255 = local write "Trigger Config"(w536) -> ()
                  }
                  event "Reset Error 4": Value Change {
                    n256 = event-data() -> ()  [unwired: 1 in, 1 out]
                    n257 = local write "Error Message 4"("" ("Error Message")) -> ()
                    n258 = local write "Error 4"(FALSE ("Error 4")) -> ()
                  }
                }
                n259 = Unbundle(w375) -> ("code"=w373:i32, "source"=w374:string)  [unwired: 1 out]
                n260 = Not Equal To 0?(x=w373) -> (x != 0?=w376:bool)
                n261 = case shown="True" w376 {
                  selector: w376 -> [_ w380]
                  tunnel: w374 -> [_ w381]
                  frame False {
                  }
                  frame True {
                    "Error Message 4" <- w381
                    "Error 4" <- w380
                  }
                }
              }
              frame "About" {
                n262 = event shown="[0] Timeout" {
                  selector: _ -> [_ _]
                  dyn-events: _ -> [_ _]
                  timeout: 100 -> [_ _]
                  tunnel: w547 -> [w557 _]
                  tunnel: [w553 _] -> w543
                  event Timeout {
                    n263 = event-data() -> ()  [unwired: 1 in, 1 out]
                    n264 = call "getDeviceName.vi"("connection ID"=w557) -> ("error out"=w554:errorcluster, "name"=→"device name":string, "connection ID out"=w555:refnum<k5>)  [unwired: 8 in]
                    n265 = call "getLockStatus.vi"("error"=w554, "connection ID"=w555) -> ("error out"=w553:errorcluster, "authorized"=w552:bool, "locked"=w551:bool)  [unwired: 6 in, 1 out]
                    n266 = case shown="True" w552 {
                      selector: w552 -> [_ w559]
                      tunnel: w551 -> [_ w558]
                      frame False {
                      }
                      frame True {
                        "authorized\nStatus" <- w559
                        "locked\nStatus" <- w558
                      }
                    }
                  }
                  event "Reset Error 8": Value Change {
                    n267 = event-data() -> ()  [unwired: 1 in, 1 out]
                    n268 = local write "Error 7"(FALSE ("Error 7")) -> ()
                    n269 = local write "Error Message 7"("" ("Error Message 9")) -> ()
                  }
                }
                n270 = Unbundle(w543) -> ("code"=w546:i32, "source"=w544:string)  [unwired: 1 out]
                n271 = Not Equal To 0?(x=w546) -> (x != 0?=w545:bool)
                n272 = case shown="True" w545 {
                  selector: w545 -> [_ w550]
                  tunnel: w544 -> [_ w549]
                  frame False {
                  }
                  frame True {
                    "Error Message 7" <- w549
                    "Error 7" <- w550
                  }
                }
              }
            }
          }
        }
        frame #2 {
          # "Exit / Disconnect"
          n273 = local write "stop"(FALSE ("stop")) -> ()
          n274 = call "close_connection.vi"("connection ID"=w562) -> ()  [unwired: 6 in, 1 out]
        }
      }
    }
  }
